vi "test Block Operations.vi"(8 "error in (no error)":errorcluster, 11 "TestCase in":refnum<class "Test_Blob.lvclass">) -> (0 "error out":errorcluster, 3 "TestCase out":refnum<class "Test_Blob.lvclass">)   [LabVIEW 2015, in "Test_Blob.lvclass"]
uses:
  Test_Blob.lvclass
  Global Parameters.vi
  Core/Session/Session.lvclass
  Blob Storage/NI_Azure_Blob.lvlib
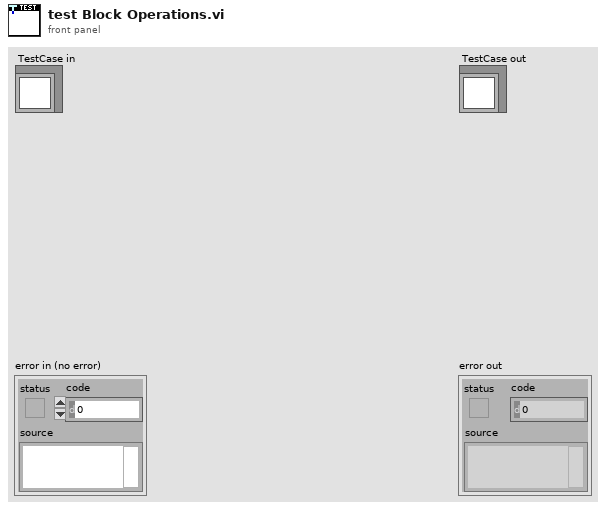
[diagram p1: front panel]
types:
  T1 = typedef "NI_Azure_Core.lvlib/Session.lvclass/Azure Credentials.ctl" = cluster{"Storage Account Name":string, "Access Key":string}
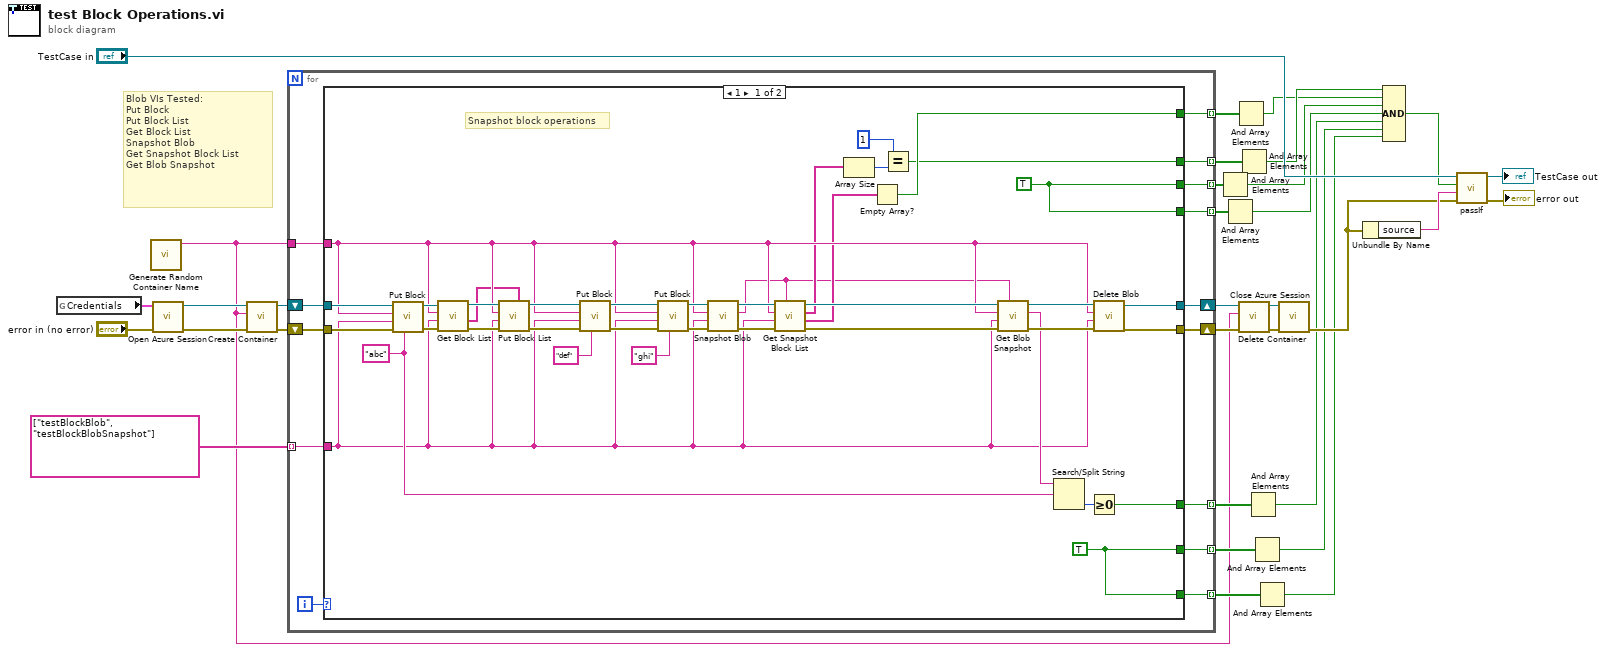
[diagram p0: block diagram]
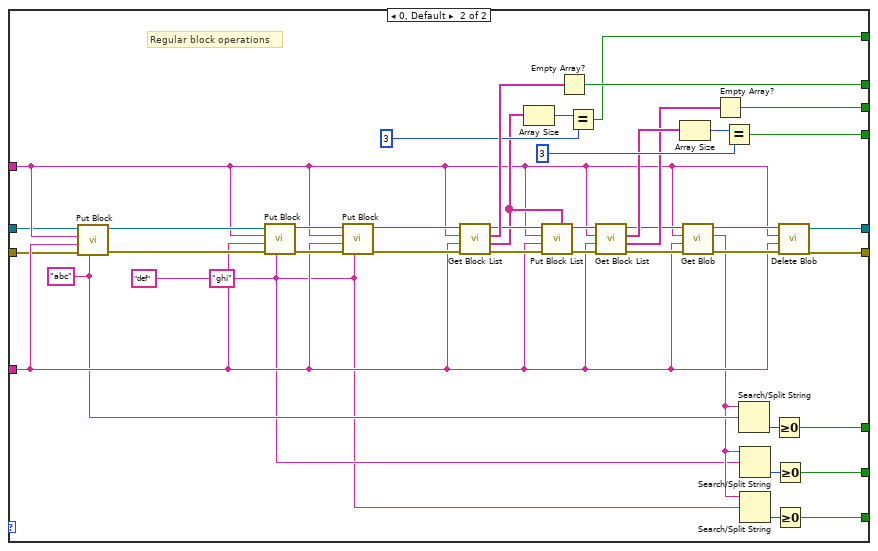
[diagram p2: hidden frame]
diagram:
  # "Blob VIs Tested:\nPut Block\nPut Block List\nGet Block List\nSnapshot Blob\nGet Snapshot Block List\nGet Blob Snapshot"
  n1 = global read "Global Parameters.vi" "Credentials"() -> (w27:T1)
  n2 = call "Generate Random Container Name.vi"() -> ("Random Container Name"=w1:string)  [unwired: 11 in]
  n3 = call "Open Azure Session.vi"("error in (no error)"="error in (no error)", "Credentials"=w27) -> ("error out"=w4:errorcluster, "Azure Session"=w6:refnum<class "Session.lvclass">)  [unwired: 8 in]
  n4 = call "Create Container.vi"("error in (no error)"=w4, "Container"=w1, "Azure Session in"=w6) -> ("error out"=w3:errorcluster, "Azure Session out"=w5:refnum<class "Session.lvclass">)  [unwired: 7 in]
  n5 = for {
    tunnel: [w42] -> w20 mode=indexing
    tunnel: [w41] -> w19 mode=indexing
    tunnel: w1 -> [w40]
    tunnel: string[] ["testBlockBlob", "testBlockBlobSnapshot"] -> [w39] mode=indexing
    tunnel: [w38] -> w18 mode=indexing
    tunnel: [w37] -> w17 mode=indexing
    tunnel: [w36] -> w16 mode=indexing
    tunnel: [w35] -> w15 mode=indexing
    tunnel: [w34] -> w14 mode=indexing
    shift-right: [w43] -> w22
    shift-left: w3 -> [w46]
    shift-right: [w44] -> w23
    shift-left: w5 -> [w45]
    i -> [w33]
    n6 = case shown="1" w33 {
      tunnel: w46 -> [w68 w85]
      tunnel: w45 -> [w69 w86]
      tunnel: [w83 w125] -> w44
      tunnel: [w82 w124] -> w43
      tunnel: [w49 w116] -> w42
      tunnel: [w53 w113] -> w41
      tunnel: w40 -> [w58 w100]
      tunnel: w39 -> [w57 w99]
      tunnel: [w55 w98] -> w38
      tunnel: [w55 w97] -> w37
      tunnel: [w70 w89] -> w36
      tunnel: [w47 w88] -> w35
      tunnel: [w47 w87] -> w34
      frame 1 {
        w47 = TRUE
        w55 = TRUE
        w75 = "abc" ("Block Content")
        # "Snapshot block operations"
        n7 = call "Put Block.vi"("Block Content"=w75, "error in (no error)"=w68, "Blob"=w57, "Container"=w58, "Azure Session in"=w69) -> ("error out"=w84:errorcluster, "Azure Session out"=w60:refnum<class "Session.lvclass">)  [unwired: 5 in]
        n8 = call "Get Block List.vi"("error in (no error)"=w84, "Blob"=w57, "Container"=w58, "Azure Session in"=w60) -> ("error out"=w61:errorcluster, "Uncommitted Blocks"=w56:string[], "Azure Session out"=w59:refnum<class "Session.lvclass">)  [unwired: 4 in, 1 out]
        n9 = call "Put Block List.vi"("Uncommitted Blocks"=w56, "error in (no error)"=w61, "Blob"=w57, "Container"=w58, "Azure Session in"=w59) -> ("error out"=w63:errorcluster, "Azure Session out"=w62:refnum<class "Session.lvclass">)  [unwired: 5 in]
        n10 = call "Put Block.vi"("Block Content"="def", "error in (no error)"=w63, "Blob"=w57, "Container"=w58, "Azure Session in"=w62) -> ("error out"=w80:errorcluster, "Azure Session out"=w81:refnum<class "Session.lvclass">)  [unwired: 5 in]
        n11 = call "Put Block.vi"("Block Content"="ghi", "error in (no error)"=w80, "Blob"=w57, "Container"=w58, "Azure Session in"=w81) -> ("error out"=w67:errorcluster, "Azure Session out"=w65:refnum<class "Session.lvclass">)  [unwired: 5 in]
        n12 = call "Snapshot Blob.vi"("error in (no error)"=w67, "Blob"=w57, "Container"=w58, "Azure Session in"=w65) -> ("error out"=w66:errorcluster, "Snapshot"=w48:string, "Azure Session out"=w64:refnum<class "Session.lvclass">)  [unwired: 5 in]
        n13 = call "Get Snapshot Block List.vi"("Snapshot"=w48, "error in (no error)"=w66, "Blob"=w57, "Container"=w58, "Azure Session in"=w64) -> ("error out"=w79:errorcluster, "Uncommitted Blocks"=w54:string[], "Committed Blocks"=w52:string[], "Azure Session out"=w78:refnum<class "Session.lvclass">)  [unwired: 3 in]
        n14 = Array Size(array=w52) -> (size(s)=w51:i32)
        n15 = Empty Array?(array=w54) -> (empty?=w53:bool)
        n16 = Equal?(x=1, y=w51) -> (x = y?=w49:bool)
        n17 = call "Get Blob Snapshot.vi"("Snapshot"=w48, "error in (no error)"=w79, "Blob"=w57, "Container"=w58, "Azure Session in"=w78) -> ("error out"=w77:errorcluster, "Blob Content"=w73:string, "Azure Session out"=w76:refnum<class "Session.lvclass">)  [unwired: 4 in]
        n18 = Search/Split String(string=w73, search string/char (-)=w75) -> (offset of match=w74:i32)  [unwired: 1 in, 2 out]
        n19 = Greater Or Equal To 0?(x=w74) -> (x >= 0?=w70:bool)
        n20 = call "Delete Blob.vi"("error in (no error)"=w77, "Blob"=w57, "Container"=w58, "Azure Session in"=w76) -> ("error out"=w82:errorcluster, "Azure Session out"=w83:refnum<class "Session.lvclass">)  [unwired: 6 in]
      }
      frame 0, Default {
        w90 = "ghi" ("Block Content")
        w91 = "def" ("Block Content")
        w96 = "abc" ("Block Content")
        # "Regular block operations"
        n21 = call "Put Block.vi"("Block Content"=w96, "error in (no error)"=w85, "Blob"=w99, "Container"=w100, "Azure Session in"=w86) -> ("error out"=w126:errorcluster, "Azure Session out"=w123:refnum<class "Session.lvclass">)  [unwired: 5 in]
        n22 = call "Put Block.vi"("Block Content"=w91, "error in (no error)"=w126, "Blob"=w99, "Container"=w100, "Azure Session in"=w123) -> ("error out"=w121:errorcluster, "Azure Session out"=w122:refnum<class "Session.lvclass">)  [unwired: 5 in]
        n23 = call "Put Block.vi"("Block Content"=w90, "error in (no error)"=w121, "Blob"=w99, "Container"=w100, "Azure Session in"=w122) -> ("error out"=w119:errorcluster, "Azure Session out"=w120:refnum<class "Session.lvclass">)  [unwired: 5 in]
        n24 = call "Get Block List.vi"("error in (no error)"=w119, "Blob"=w99, "Container"=w100, "Azure Session in"=w120) -> ("error out"=w118:errorcluster, "Uncommitted Blocks"=w110:string[], "Committed Blocks"=w117:string[], "Azure Session out"=w111:refnum<class "Session.lvclass">)  [unwired: 4 in]
        n25 = Array Size(array=w110) -> (size(s)=w115:i32)
        n26 = call "Put Block List.vi"("Uncommitted Blocks"=w110, "error in (no error)"=w118, "Blob"=w99, "Container"=w100, "Azure Session in"=w111) -> ("error out"=w112:errorcluster, "Azure Session out"=w108:refnum<class "Session.lvclass">)  [unwired: 5 in]
        n27 = Empty Array?(array=w117) -> (empty?=w116:bool)
        n28 = Equal?(x=w115, y=3) -> (x = y?=w113:bool)
        n29 = call "Get Block List.vi"("error in (no error)"=w112, "Blob"=w99, "Container"=w100, "Azure Session in"=w108) -> ("error out"=w109:errorcluster, "Uncommitted Blocks"=w104:string[], "Committed Blocks"=w105:string[], "Azure Session out"=w102:refnum<class "Session.lvclass">)  [unwired: 4 in]
        n30 = Array Size(array=w105) -> (size(s)=w106:i32)
        n31 = call "Get Blob.vi"("error in (no error)"=w109, "Blob"=w99, "Container"=w100, "Azure Session in"=w102) -> ("error out"=w103:errorcluster, "Blob Content"=w92:string, "Azure Session out"=w101:refnum<class "Session.lvclass">)  [unwired: 5 in]
        n32 = Empty Array?(array=w104) -> (empty?=w98:bool)
        n33 = Equal?(x=w106, y=3) -> (x = y?=w97:bool)
        n34 = Search/Split String(string=w92, search string/char (-)=w96) -> (offset of match=w95:i32)  [unwired: 1 in, 2 out]
        n35 = Search/Split String(string=w92, search string/char (-)=w91) -> (offset of match=w94:i32)  [unwired: 1 in, 2 out]
        n36 = Search/Split String(string=w92, search string/char (-)=w90) -> (offset of match=w93:i32)  [unwired: 1 in, 2 out]
        n37 = Greater Or Equal To 0?(x=w95) -> (x >= 0?=w89:bool)
        n38 = Greater Or Equal To 0?(x=w94) -> (x >= 0?=w88:bool)
        n39 = Greater Or Equal To 0?(x=w93) -> (x >= 0?=w87:bool)
        n40 = call "Delete Blob.vi"("error in (no error)"=w103, "Blob"=w99, "Container"=w100, "Azure Session in"=w101) -> ("error out"=w124:errorcluster, "Azure Session out"=w125:refnum<class "Session.lvclass">)  [unwired: 6 in]
      }
    }
  }
  n41 = And Array Elements(Boolean array=w18) -> (logical AND=w9:bool)
  n42 = And Array Elements(Boolean array=w17) -> (logical AND=w10:bool)
  n43 = And Array Elements(Boolean array=w19) -> (logical AND=w7:bool)
  n44 = And Array Elements(Boolean array=w20) -> (logical AND=w8:bool)
  n45 = call "Delete Container.vi"("error in (no error)"=w22, "Container"=w1, "Azure Session in"=w23) -> ("error out"=w26:errorcluster, "Azure Session out"=w24:refnum<class "Session.lvclass">)  [unwired: 7 in]
  n46 = And Array Elements(Boolean array=w16) -> (logical AND=w11:bool)
  n47 = And Array Elements(Boolean array=w15) -> (logical AND=w12:bool)
  n48 = And Array Elements(Boolean array=w14) -> (logical AND=w13:bool)
  n49 = call "Close Azure Session.vi"("error in (no error)"=w26, "Azure Session"=w24) -> ("error out"=w25:errorcluster)  [unwired: 9 in]
  n50 = Unbundle By Name(w25) -> ("source"=w29:string)
  n51 = Compound Arithmetic op=AND(w8, w7, w9, w10, w11, w12, w13) -> (w21:bool)
  n52 = call-dynamic "passIf.vi"("error in (no error)"=w25, "message (\"\")"=w29, "pass"=w21, "TestCase in"="TestCase in") -> ("error out"=→"error out":errorcluster, "TestCase out"=→"TestCase out":refnum<class "Test_Blob.lvclass">)  [unwired: 6 in]
